vi "Create.vi"(8 "error in (no error)":errorcluster) -> (0 "error out":errorcluster, 3 "Default Buffer Converter Component":refnum<class "Default Buffer Converter Component.lvclass">)   [LabVIEW 2020, in "DSF Core.lvlib" / "Default Buffer Converter Component.lvclass"]
uses:
  Default Buffer Converter Component.lvclass
  C:/Users/nitest/Desktop/Git/niveristand-data-sharing-framework-custom-device/Source/Core/Classes/Component/Component.lvclass
  Components/Buffer Converters/DSF Type Converter/Default Buffer Converter.lvclass
  Components/Buffer Converters/DSF Type Converter/User Interfaces/Default Buffer Converter User Interfaces.lvclass
  Components/Buffer Converters/DSF Type Converter/Configurations/Default Buffer Converter Configurations.lvclass
  Component.lvclass/Component.ctl
  Component Configuration/Find.vi
  Component User Interface/Find.vi
  <vilib>/Utility/error.llb/Clear Errors.vi
  Component User Interface/Component User Interfaces.lvclass
  Component Configuration/Component Configurations.lvclass
  Component.lvclass
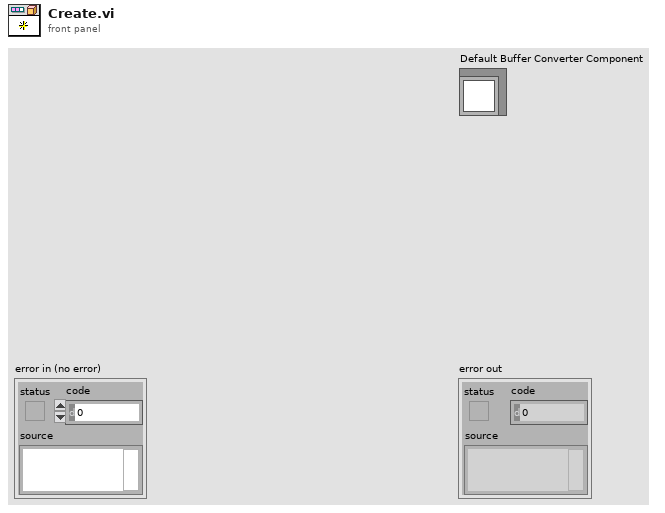
[diagram p1: front panel]
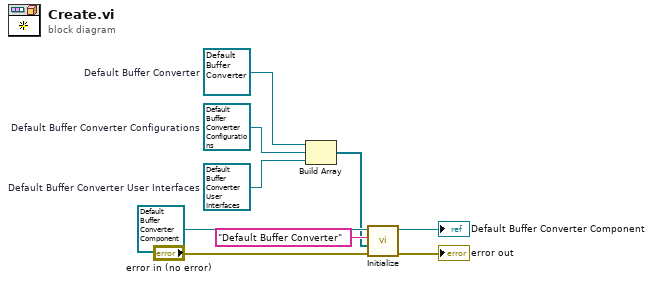
[diagram p0: block diagram]
diagram:
  w1 = refnum<class "Default Buffer Converter.lvclass"> refnum  # Default Buffer Converter
  w4 = refnum<class "Default Buffer Converter User Interfaces.lvclass"> refnum  # Default Buffer Converter User Interfaces
  w3 = refnum<class "Default Buffer Converter Configurations.lvclass"> refnum  # Default Buffer Converter Configurations
  n1 = Build Array(w1, w3, w4) -> (w2:refnum<class>[])
  n2 = call "Initialize.vi"("error in (no error)"="error in (no error)", "objects"=w2, "name"="Default Buffer Converter", "Component in"=refnum<class "Default Buffer Converter Component.lvclass"> refnum ("Default Buffer Converter Component in")) -> ("error out"=→"error out":errorcluster, "Component out"=→"Default Buffer Converter Component":refnum<class "Default Buffer Converter Component.lvclass">)  [unwired: 6 in]
